vi "GTcode_v6.vi"() -> ()   [LabVIEW 2016]
uses:
  <vilib>/Utility/config.llb/Write Key (String).vi
  <vilib>/Utility/config.llb/Write Key (U32).vi
  <vilib>/Utility/config.llb/Write Key (Double).vi
  <vilib>/Utility/config.llb/Write Key (I32).vi
  <vilib>/Utility/config.llb/Read Key (U32).vi
  <vilib>/Utility/config.llb/Read Key (I32).vi
  DCScode_simulISS_MAP/flex05-4chPascal.dll
  <vilib>/Utility/config.llb/NI_LVConfig.lvlib
  DCScode_simulISS_MAP/flex05oem8chauto100nsPASCAL_win7.dll
  <vilib>/Analysis/NI_AALBase.lvlib
panel:
  in  "Tab Control":T1(tab)=enum."Real Time Fitting Parameters"
  out "mean":dbl format="%0.1e"
  out "COV":dbl format="%0.1f"
  in  "Fixed Time":bool
  in  "Detector Used":T2(ring)=enum."Det 2"
  in  "Real Time Fitting?":bool=TRUE
  out "g2":cluster{"Delay Time":sgl[], sgl[]}[](graph) caption="Normalized Correlation Function"
  out "Tau":cluster{"tmp":dbl, dbl}(graph) caption="Relative Changes of Flow"
  in  "QUIT":bool
  in  "Clear plots":bool
  in  "Baseline":bool
  in  "MARK\nMark":bool
  in  "Stop":bool
  in  "Sequence Scan":bool
  out "Mark #":u32
  out "Trial #":u32
  out "Frame #":u32
  out "Det 8":sgl format="%.3f"
  out "Det 7":sgl format="%.3f"
  out "Det 6":sgl format="%.3f"
  out "Det 5":sgl format="%.3f"
  out "Det 4":sgl format="%.3f"
  out "Det 3":sgl format="%.3f"
  out "Det 2":sgl format="%.3f"
  out "Det 1":sgl format="%.3f"
  out "Computer Time":string="2010-1-12 23:16:10"
  in  "D1":bool
  in  "D2":bool
  in  "D3":bool
  in  "D4":bool
  in  "D5":bool
  in  "D6":bool
  in  "D7":bool
  in  "D8":bool
  out "Tau 2":T3(graph)={1.6593152555505744e-08, 3.9427894777554196e-08, 4.065716407938411e-08, 1.5135790977358522e-08, 2.4870420100428357e-08, 7.094765128107397e-08, 0.0, 4.1348620928852906e-07, 1.5886917674344795e-08, 4.0280526032721455e-08, -1.0, -1.0} caption="Blood Flow Index (cm2/s)"
  in  "Fixed # of Frames":u32=5
  out "Status":string="Quit"
  in  "Optical Switch OPEN":bool
  in  "Delay between frames(ms)":u32=500
  out "Time Left (ms)":sgl format="%.3f"
  in  "Integration Time (ms)":sgl=1000.0 min=1 max=13000 step=1
  in  "File\nName:":string="test0"
  in  "Data Save Directory:":path=path "C:/data"
  in  "ISS Lasers ON":bool
  in  "Test":bool
  in  "Lines":tag="Dev1/port1/line0:1, Dev1/port1/line3:7"
  in  "Delaytime(ms)":u32=200
  in  "Initialize Correlator":bool
  in  "Detector Select":enum32{"4 Detectors", "8 Detectors"}(radio)=enum."8 Detectors"
  in  "Update Time (ms)\nDO NOT CHANGE!":u32=105 min=1 max=999 step=1
  in  "Laser Input Name":refnum<visa-resource-name>="COM7"
  out "Flow in each detector":dbl[](array[numeric])=[-1.0, -1.0, -1.0, -1.0, -1.0, -1.0, -1.0, -1.0, -1.0, -1.0, -1.0, -1.0]
  in  "Visible Averages":bool[](array[boolean])=[FALSE, FALSE, FALSE, FALSE]
  in  "Avg":bool[][](array[boolean])=[[FALSE, FALSE, FALSE, FALSE, FALSE, FALSE, FALSE, FALSE], [FALSE, FALSE, FALSE, FALSE, FALSE, FALSE, FALSE, FALSE], [FALSE, FALSE, FALSE, FALSE, FALSE, FALSE, FALSE, FALSE], [FALSE, FALSE, FALSE, FALSE, FALSE, FALSE, FALSE, FALSE]]
  in  "rho":dbl[](array[numeric])=[2.5, 2.5, 2.5, 2.5, 2.5, 2.5, 2.5, 2.5, -1.0, -1.0, -1.0, -1.0]
  in  "Other Settings":u32[](array[numeric])=[1, 120, 0, 1] caption="Flow in each detector"
  in  "Initial Guess":dbl[](array[numeric])=[1e-08, 0.5, 0.05, 10.0] caption="Flow in each detector"
  out "4CH?":bool
  out "Detector#":u32=1
  out "Source#":u32=1
  # "kHz"
  # "kHz"
  # "Don't Change these Parameters unless you know clearly what you are doing"
  # "ISS Triggers Setup"
  # "Channel Parameters"
  # "Step1"
  # "Line"
  # "0"
  # "1"
  # "3"
  # "4"
  # "5"
  # "6"
  # "7"
  # "*The number of lines in the list must\nmatch the number of elements in\nthe array."
  # "Step2"
  # "Line"
  # "0"
  # "1"
  # "3"
  # "4"
  # "5"
  # "6"
  # "7"
  # "Step3"
  # "Line"
  # "0"
  # "1"
  # "3"
  # "4"
  # "5"
  # "6"
  # "7"
  # "Line    Signal\n\n0           ISS Trigger (0: OFF, 1: ON)\n1           Flow Laser 1 ON/OFF (0:OFF, 1:ON)\n2           ISS Data Acquisition (0: DONE, 1: NO)\n3           ISS Laser ON/OFF (0: ON, 1: OFF)\n4           Trigger for Marks  (0: OFF, 1: ON)\n5           Flow Laser 2 ON/OFF (0:OFF, 1:ON)\n6           Reserved\n7           Reserved"
  # "Wait ISS Data Acuisition DONE Signal"
  # "Step4"
  # "Step5"
  # "Line"
  # "0"
  # "1"
  # "3"
  # "4"
  # "5"
  # "6"
  # "7"
  # "Flow Lasers Setup"
  # "FROM FRONT PANEL"
  # "Line"
  # "0"
  # "1"
  # "3"
  # "4"
  # "5"
  # "6"
  # "7"
  # "Line"
  # "0"
  # "1"
  # "3"
  # "4"
  # "5"
  # "6"
  # "7"
  # "Det 1"
  # "Det 2"
  # "Det 3"
  # "Det 4"
  # "Det 5"
  # "Det 6"
  # "Det 7"
  # "Det 8"
  # "Avg 1"
  # "Avg 2"
  # "Avg 3"
  # "Avg 4"
  # "Db"
  # "Beta"
  # "Mua"
  # "MuS'"
  # "1"
  # "2"
  # "3"
  # "4"
  # "5"
  # "6"
  # "7"
  # "8"
  # "Avg 1"
  # "Starting Pt"
  # "End Pt"
  # "Approximate"
  # "Variables"
  # "Avg 2"
  # "Avg 3"
  # "Avg 4"
  # "Source Detector  Separations"
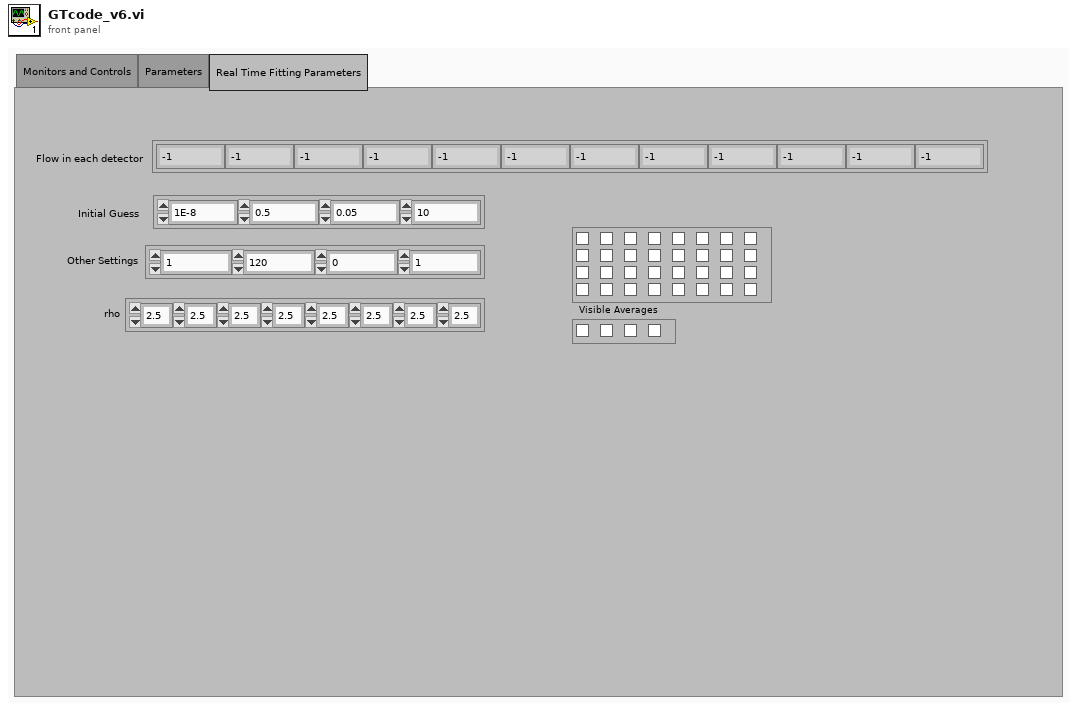
[diagram p1: front panel]
types:
  T1 = enum32{"Monitors and Controls", "Parameters", "Real Time Fitting Parameters"}
  T2 = enum16{"Det 1", "Det 2", "Det 3", "Det 4", "Det 5", "Det 6", "Det 7", "Det 8"}
  T3 = cluster{dbl, dbl, dbl, dbl, dbl, dbl, dbl, dbl, dbl, dbl, dbl, dbl}
  T4 = enum8{"Enabled", "Disabled", "Disabled and Grayed Out"}
  T5 = cluster{dbl, dbl, dbl, dbl, dbl, dbl, dbl, dbl, dbl, dbl, dbl, dbl}[]
  T6 = typedef "NI_LVConfig.lvlib/Config Data RefNum.ctl" = refnum<k1>
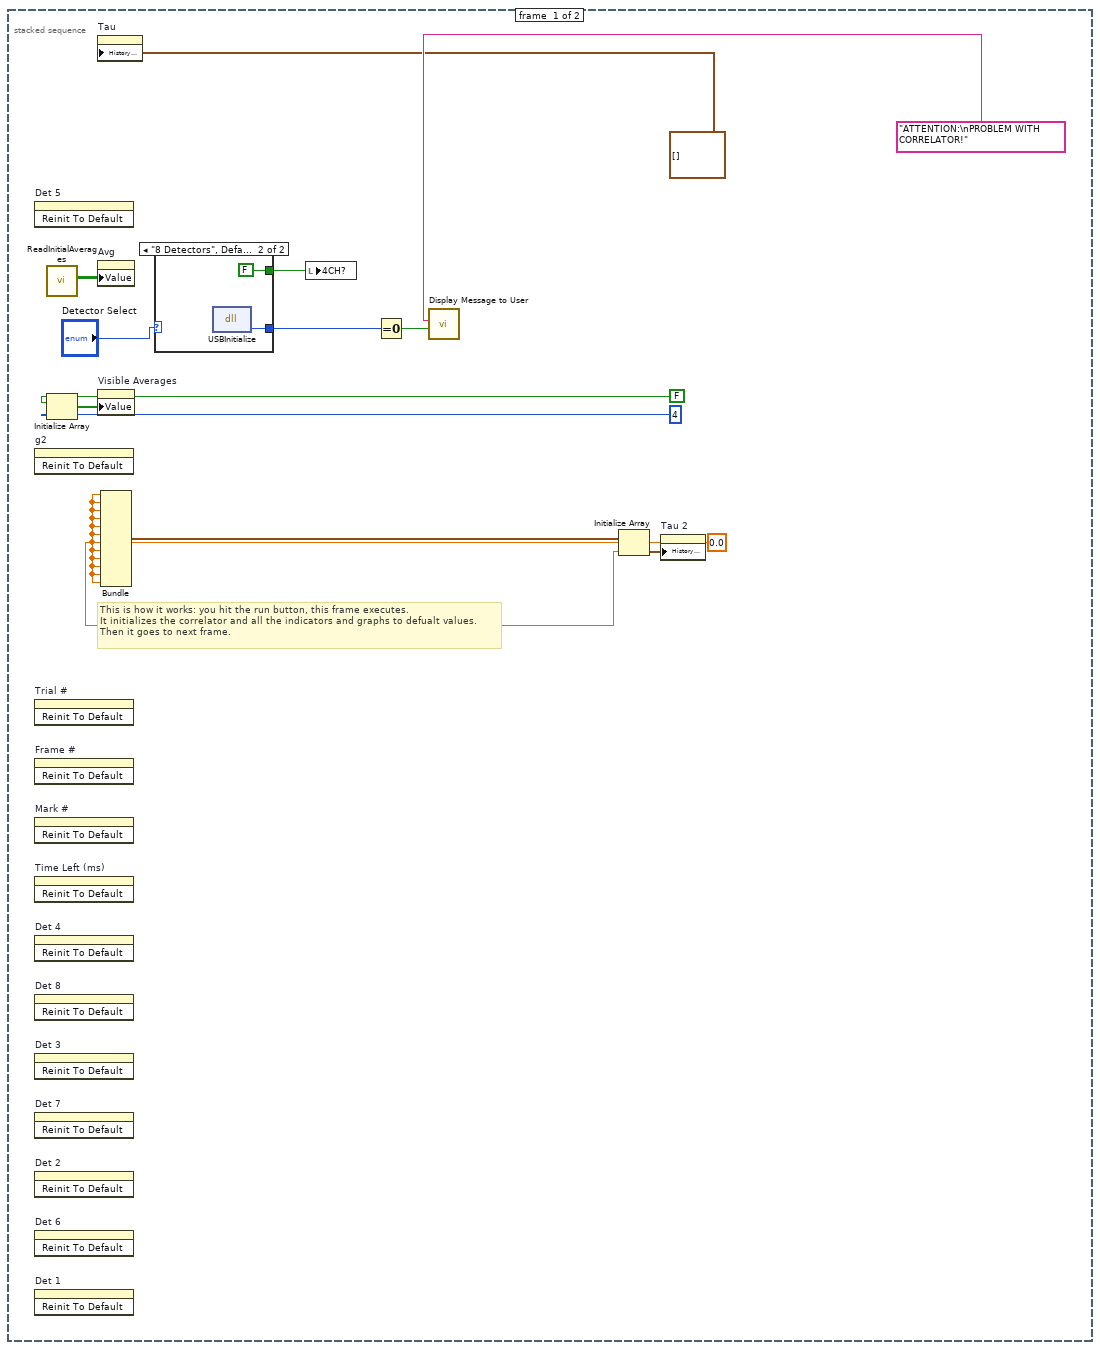
[diagram p2: hidden frame]
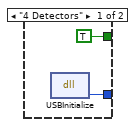
[diagram p3: hidden frame]
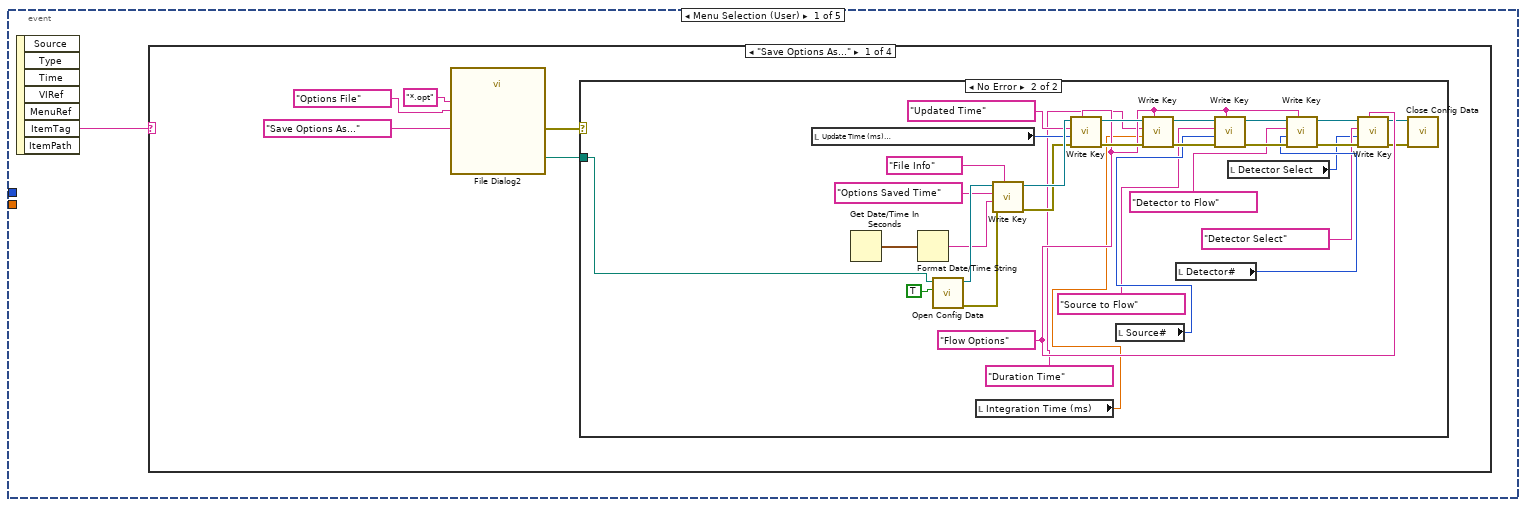
[diagram p5: hidden frame]
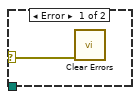
[diagram p6: hidden frame]
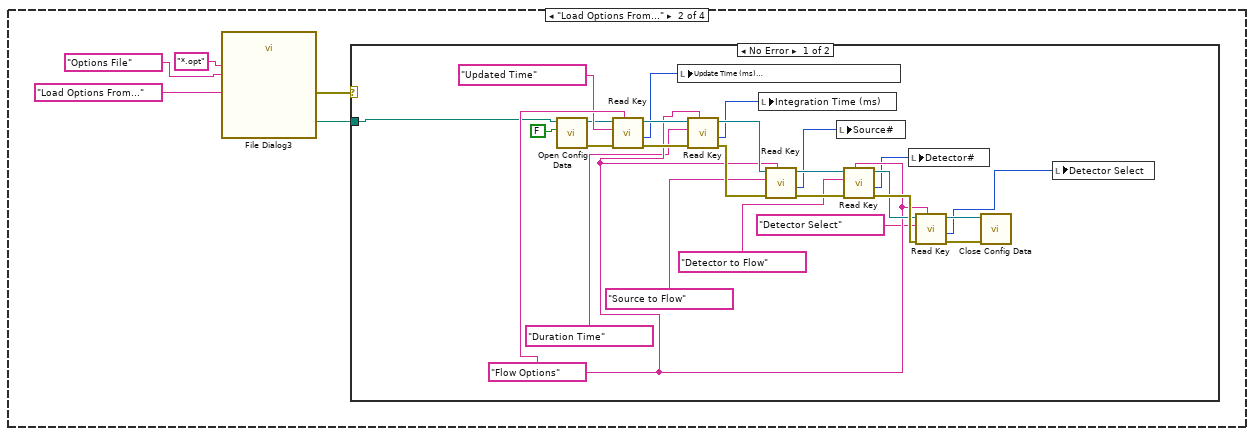
[diagram p7: hidden frame]
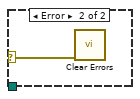
[diagram p8: hidden frame]
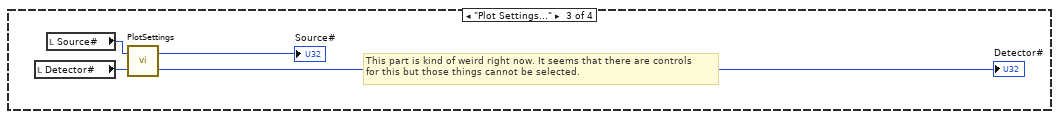
[diagram p9: hidden frame]
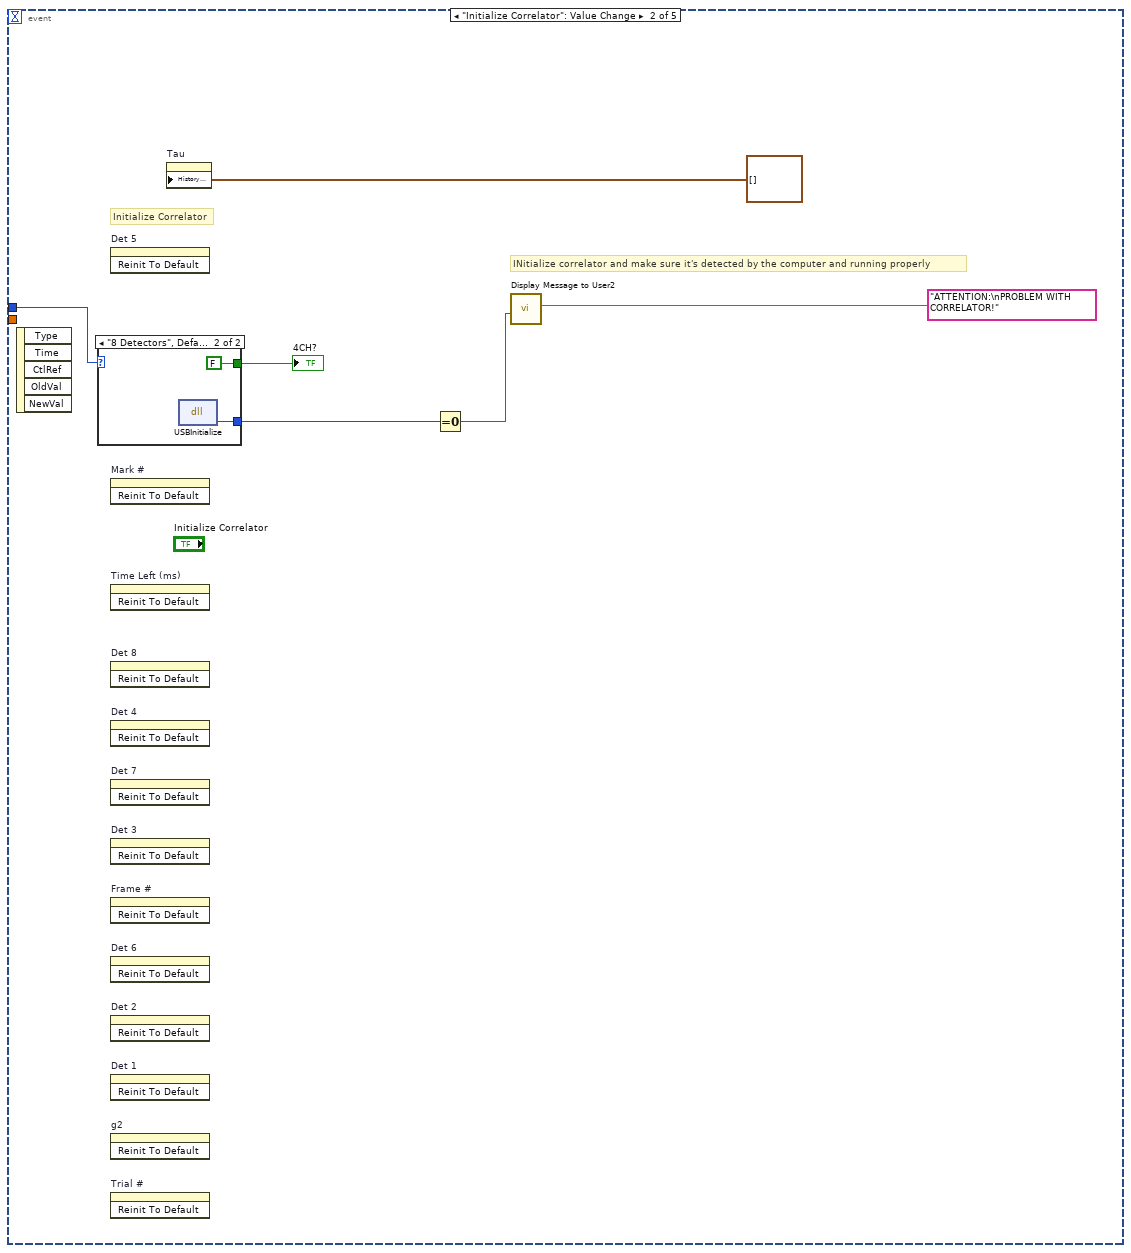
[diagram p11: hidden frame]
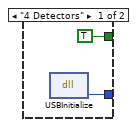
[diagram p12: hidden frame]
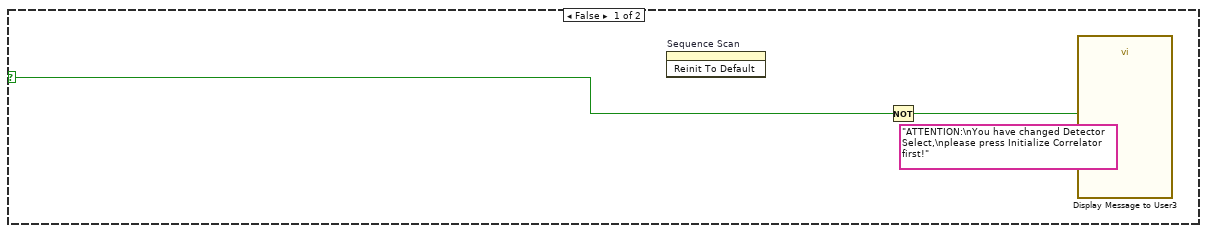
[diagram p13: hidden frame]
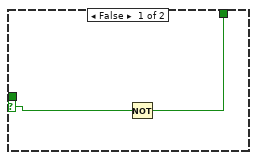
[diagram p14: hidden frame]
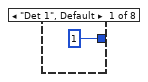
[diagram p20: hidden frame]
diagram:
  n1 = local read "Laser Input Name"() -> (w1:refnum<visa-resource-name>)
  n2 = call "iBs.vi"("Laser On/Off"=FALSE, "VISA resource name"=w1) -> ()
  n3 = stacked-sequence {
    frame #0 {
      w5 = 0.0
      # "This is how it works: you hit the run button, this frame executes.\nIt initializes the correlator and all the indicators and graphs to defualt values.\nThen it goes to next frame."
      n4 = invoke on="Det 5" class="DigNum (strict)" method="Reinit To Default"() -> ()  [unwired: 3 in, 3 out]
      n5 = invoke on="g2" class="XYGraph (strict)" method="Reinit To Default"() -> ()  [unwired: 3 in, 3 out]
      n6 = invoke on="Trial #" class="DigNum (strict)" method="Reinit To Default"() -> ()  [unwired: 3 in, 3 out]
      n7 = invoke on="Frame #" class="DigNum (strict)" method="Reinit To Default"() -> ()  [unwired: 3 in, 3 out]
      n8 = invoke on="Mark #" class="DigNum (strict)" method="Reinit To Default"() -> ()  [unwired: 3 in, 3 out]
      n9 = invoke on="Time Left (ms)" class="DigNum (strict)" method="Reinit To Default"() -> ()  [unwired: 3 in, 3 out]
      n10 = invoke on="Det 4" class="DigNum (strict)" method="Reinit To Default"() -> ()  [unwired: 3 in, 3 out]
      n11 = invoke on="Det 8" class="DigNum (strict)" method="Reinit To Default"() -> ()  [unwired: 3 in, 3 out]
      n12 = invoke on="Det 3" class="DigNum (strict)" method="Reinit To Default"() -> ()  [unwired: 3 in, 3 out]
      n13 = invoke on="Det 7" class="DigNum (strict)" method="Reinit To Default"() -> ()  [unwired: 3 in, 3 out]
      n14 = invoke on="Det 2" class="DigNum (strict)" method="Reinit To Default"() -> ()  [unwired: 3 in, 3 out]
      n15 = invoke on="Det 6" class="DigNum (strict)" method="Reinit To Default"() -> ()  [unwired: 3 in, 3 out]
      n16 = invoke on="Det 1" class="DigNum (strict)" method="Reinit To Default"() -> ()  [unwired: 3 in, 3 out]
      n17 = call "ReadInitialAverages.vi"() -> ("avgOut"=w4:bool[][])  [unwired: 11 in]
      n18 = Initialize Array(FALSE, 4) -> (w3:bool[])
      n19 = property on="Tau" class="WFChart (strict)"("History Data"=cluster{"tmp":dbl, dbl}[] []) -> ()  [unwired: 2 in, 2 out]
      n20 = property on="Avg" class="Arr (strict)"("Value"=w4) -> ()  [unwired: 2 in, 2 out]
      n21 = property on="Visible Averages" class="Arr (strict)"("Value"=w3) -> ()  [unwired: 2 in, 2 out]
      n22 = Bundle(w5, w5, w5, w5, w5, w5, w5, w5, w5, w5, w5, w5) -> (w7:T3)  [unwired: 1 in]
      n23 = case shown="\"8 Detectors\", Default" "Detector Select" {
        tunnel: [w17 w19] -> w15
        tunnel: [TRUE FALSE] -> w13
        frame "4 Detectors" {
          n24 = dll-call lib="C:/Users/BUCKLEY-ADMIN/Desktop/DCScode_simulISS_MAP/flex05-4chPascal.dll" fn="USBInitialize" label="InitCH4"() -> ("return type"=w17:u8)  [unwired: 3 in, 2 out]
        }
        frame "8 Detectors", Default {
          n25 = dll-call lib="C:/Users/BUCKLEY-ADMIN/Desktop/DCScode_simulISS_MAP/flex05oem8chauto100nsPASCAL_win7.dll" fn="USBInitialize" label="InitCH8"() -> ("return type"=w19:u8)  [unwired: 3 in, 2 out]
        }
      }
      n26 = local write "4CH?"(w13) -> ()
      n27 = Equal To 0?(x=w15) -> (x = 0?=w14:bool)
      n28 = call "Display Message to User"("Enable"=w14, "Message"="ATTENTION:\nPROBLEM WITH CORRELATOR!") -> ()  [unwired: 8 in, 2 out]
      n29 = Initialize Array(w7, w5) -> (w6:T5)
      n30 = property on="Tau 2" class="WFChart (strict)"("History Data"=w6) -> ()  [unwired: 2 in, 2 out]
    }
    frame #1 {
      n31 = while {
        stop <- w23 stop-if-true
        # "Looks at whether using 4 or 8 ch correlator\nGenerates time points for g2 function based on correlator"
        n32 = local read "Detector Select"() -> (w21:enum32{"4 Detectors", "8 Detectors"})
        n33 = case shown="\"8 Detectors\"" w21 {
          tunnel: [_ w24] -> w20
          frame "4 Detectors", Default {
          }
          frame "8 Detectors" {
            n34 = formula code="int i,j;\nfloat DelayTime[256];\nfloat first_delay;\n\nfirst_delay = 2E-7;\n\nfor(i=0;i<16;i++)\nDelayTime[i] = (i+1)*first_delay;\nfor(j=1;j<31;j++)\n    for(i=0;i<8;i++)\n         DelayTime[i+(j-1)*8+16] = DelayTime[(j-1)*8+16+i-1]+first_delay*pow(2,j);"() -> ("DelayTime"=w24:dbl[])
          }
        }
        n35 = event shown="[2] \"Sequence Scan\": Value Change" {
          selector: _ -> [_ _ _ _ _]
          dyn-events: _ -> [_ _ _ _ _]
          timeout: 500 -> [_ _ _ _ _]
          tunnel: w20 -> [_ _ w114 _ _]
          tunnel: [_ _ _ "QUIT" _] -> w23
          tunnel: w21 -> [_ w101 w110 w598 _]
          event Menu Selection (User) {
            n36 = event-data() -> ("ItemTag"=w25:string)  [unwired: 1 in, 6 out]
            n37 = case shown="\"Save Options As...\"" w25 {
              frame "Save Options As..." {
                n38 = call "File Dialog2"("prompt"="Save Options As...", "pattern (all files)"="*.opt", "pattern label"="Options File") -> ("selected path"=w27:path, "error out"=w26:errorcluster)  [unwired: 9 in, 2 out]
                n39 = case shown="No Error" w26 {
                  selector: w26 -> [w31 _]
                  tunnel: w27 -> [_ w62]
                  frame Error {
                    n40 = call <vilib>:"Clear Errors.vi"("error in (no error)"=w31) -> ()  [unwired: 5 in, 2 out]
                  }
                  frame No Error {
                    w49 = "Flow Options"
                    n41 = local read "Update Time (ms)\nDO NOT CHANGE!"() -> (w42:u32)
                    n42 = Get Date/Time In Seconds() -> (seconds since 1Jan1904=w48:timestamp)
                    n43 = Format Date/Time String(seconds (now)=w48) -> (date/time string=w44:string)  [unwired: 2 in]
                    n44 = call <vilib>:"Open Config Data.vi"("create file if necessary (T)"=TRUE, "configuration file path"=w62) -> ("error out"=w60:errorcluster, "refnum"=w59:T6)  [unwired: 7 in, 1 out]
                    n45 = local read "Integration Time (ms)"() -> (w40:sgl)
                    n46 = call-poly <vilib>:"Write Key.vi"("section"="File Info", "error in (no error)"=w60, "value"=w44, "key"="Options Saved Time", "refnum"=w59) -> ("error out"=w46:errorcluster, "refnum out"=w47:T6)  [unwired: 4 in, 1 out]
                    n47 = call-poly <vilib>:"Write Key.vi"("section"=w49, "error in (no error)"=w46, "value"=w42, "key"="Updated Time", "refnum"=w47) -> ("error out"=w58:errorcluster, "refnum out"=w57:T6)  [unwired: 4 in, 1 out]
                    n48 = local read "Source#"() -> (w39:u32)
                    n49 = call-poly <vilib>:"Write Key.vi"("section"=w49, "error in (no error)"=w58, "value"=w40, "key"="Duration Time", "refnum"=w57) -> ("error out"=w53:errorcluster, "refnum out"=w54:T6)  [unwired: 4 in, 1 out]
                    n50 = local read "Detector#"() -> (w36:u32)
                    n51 = call-poly <vilib>:"Write Key.vi"("section"=w49, "error in (no error)"=w53, "value"=w39, "key"="Source to Flow", "refnum"=w54) -> ("error out"=w55:errorcluster, "refnum out"=w56:T6)  [unwired: 4 in, 1 out]
                    n52 = local read "Detector Select"() -> (w34:enum32{"4 Detectors", "8 Detectors"})
                    n53 = call-poly <vilib>:"Write Key.vi"("section"=w49, "error in (no error)"=w55, "value"=w36, "key"="Detector to Flow", "refnum"=w56) -> ("error out"=w52:errorcluster, "refnum out"=w51:T6)  [unwired: 4 in, 1 out]
                    n54 = call-poly <vilib>:"Write Key.vi"("section"=w49, "error in (no error)"=w52, "value"=w34, "key"="Detector Select", "refnum"=w51) -> ("error out"=w32:errorcluster, "refnum out"=w33:T6)  [unwired: 4 in, 1 out]
                    n55 = call <vilib>:"Close Config Data.vi"("error in (no error)"=w32, "refnum"=w33) -> ()  [unwired: 8 in, 2 out]
                  }
                }
              }
              frame "Load Options From..." {
                n56 = call "File Dialog3"("prompt"="Load Options From...", "pattern (all files)"="*.opt", "pattern label"="Options File") -> ("selected path"=w64:path, "error out"=w63:errorcluster)  [unwired: 9 in, 2 out]
                n57 = case shown="No Error" w63 {
                  selector: w63 -> [_ w93]
                  tunnel: w64 -> [w68 _]
                  frame No Error {
                    w83 = "Flow Options"
                    n58 = call <vilib>:"Open Config Data.vi"("create file if necessary (T)"=FALSE, "configuration file path"=w68) -> ("error out"=w75:errorcluster, "refnum"=w74:T6)  [unwired: 7 in, 1 out]
                    n59 = call-poly <vilib>:"Read Key.vi"("section"=w83, "error in (no error)"=w75, "key"="Updated Time", "refnum"=w74) -> ("error out"=w91:errorcluster, "value"=w73:u32, "refnum out"=w90:T6)  [unwired: 4 in, 1 out]
                    n60 = local write "Update Time (ms)\nDO NOT CHANGE!"(w73) -> ()
                    n61 = call-poly <vilib>:"Read Key.vi"("section"=w83, "error in (no error)"=w91, "key"="Duration Time", "refnum"=w90) -> ("error out"=w86:errorcluster, "value"=w72:i32, "refnum out"=w87:T6)  [unwired: 4 in, 1 out]
                    n62 = local write "Integration Time (ms)"(w72) -> ()
                    n63 = call-poly <vilib>:"Read Key.vi"("section"=w83, "error in (no error)"=w86, "key"="Source to Flow", "refnum"=w87) -> ("error out"=w88:errorcluster, "value"=w69:u32, "refnum out"=w89:T6)  [unwired: 4 in, 1 out]
                    n64 = local write "Source#"(w69) -> ()
                    n65 = call-poly <vilib>:"Read Key.vi"("section"=w83, "error in (no error)"=w88, "key"="Detector to Flow", "refnum"=w89) -> ("error out"=w85:errorcluster, "value"=w70:u32, "refnum out"=w84:T6)  [unwired: 4 in, 1 out]
                    n66 = local write "Detector#"(w70) -> ()
                    n67 = call-poly <vilib>:"Read Key.vi"("section"=w83, "error in (no error)"=w85, "key"="Detector Select", "refnum"=w84) -> ("error out"=w76:errorcluster, "value"=w71:u32, "refnum out"=w77:T6)  [unwired: 4 in, 1 out]
                    n68 = call <vilib>:"Close Config Data.vi"("error in (no error)"=w76, "refnum"=w77) -> ()  [unwired: 8 in, 2 out]
                    n69 = local write "Detector Select"(w71) -> ()
                  }
                  frame Error {
                    n70 = call <vilib>:"Clear Errors.vi"("error in (no error)"=w93) -> ()  [unwired: 5 in, 2 out]
                  }
                }
              }
              frame "Plot Settings..." {
                # "This part is kind of weird right now. It seems that there are controls\nfor this but those things cannot be selected."
                n71 = local read "Detector#"() -> (w95:u32)
                n72 = local read "Source#"() -> (w96:u32)
                n73 = call "PlotSettings.vi"("Detectorin"=w95, "Sourcein"=w96) -> ("Detector#"=→"Detector#":u32, "Source#"=→"Source#":u32)
              }
              frame Default {
              }
            }
          }
          event "Initialize Correlator": Value Change {
            # "INitialize correlator and make sure it's detected by the computer and running properly"
            # "Initialize Correlator"
            n74 = event-data() -> ()  [unwired: 1 in, 5 out]
            n75 = case shown="\"8 Detectors\", Default" w101 {
              tunnel: [w105 w107] -> w103
              tunnel: [TRUE FALSE] -> w100
              frame "4 Detectors" {
                n76 = dll-call lib="C:/Users/BUCKLEY-ADMIN/Desktop/DCScode_simulISS_MAP/flex05-4chPascal.dll" fn="USBInitialize" label="InitCH4"() -> ("return type"=w105:u8)  [unwired: 3 in, 2 out]
              }
              frame "8 Detectors", Default {
                n77 = dll-call lib="C:/Users/BUCKLEY-ADMIN/Desktop/DCScode_simulISS_MAP/flex05oem8chauto100nsPASCAL_win7.dll" fn="USBInitialize" label="InitCH8"() -> ("return type"=w107:u8)  [unwired: 3 in, 2 out]
              }
            }
            "4CH?" <- w100
            n78 = invoke on="Det 5" class="DigNum (strict)" method="Reinit To Default"() -> ()  [unwired: 3 in, 3 out]
            n79 = invoke on="Mark #" class="DigNum (strict)" method="Reinit To Default"() -> ()  [unwired: 3 in, 3 out]
            n80 = invoke on="Time Left (ms)" class="DigNum (strict)" method="Reinit To Default"() -> ()  [unwired: 3 in, 3 out]
            n81 = invoke on="Det 8" class="DigNum (strict)" method="Reinit To Default"() -> ()  [unwired: 3 in, 3 out]
            n82 = invoke on="Det 4" class="DigNum (strict)" method="Reinit To Default"() -> ()  [unwired: 3 in, 3 out]
            n83 = invoke on="Det 7" class="DigNum (strict)" method="Reinit To Default"() -> ()  [unwired: 3 in, 3 out]
            n84 = invoke on="Det 3" class="DigNum (strict)" method="Reinit To Default"() -> ()  [unwired: 3 in, 3 out]
            n85 = invoke on="Frame #" class="DigNum (strict)" method="Reinit To Default"() -> ()  [unwired: 3 in, 3 out]
            n86 = invoke on="Det 6" class="DigNum (strict)" method="Reinit To Default"() -> ()  [unwired: 3 in, 3 out]
            n87 = invoke on="Det 2" class="DigNum (strict)" method="Reinit To Default"() -> ()  [unwired: 3 in, 3 out]
            n88 = invoke on="Det 1" class="DigNum (strict)" method="Reinit To Default"() -> ()  [unwired: 3 in, 3 out]
            n89 = invoke on="g2" class="XYGraph (strict)" method="Reinit To Default"() -> ()  [unwired: 3 in, 3 out]
            n90 = invoke on="Trial #" class="DigNum (strict)" method="Reinit To Default"() -> ()  [unwired: 3 in, 3 out]
            n91 = property on="Tau" class="WFChart (strict)"("History Data"=cluster{"tmp":dbl, dbl}[] []) -> ()  [unwired: 2 in, 2 out]
            n92 = Equal To 0?(x=w103) -> (x = 0?=w102:bool)
            n93 = call "Display Message to User2"("Enable"=w102, "Message"="ATTENTION:\nPROBLEM WITH CORRELATOR!") -> ()  [unwired: 8 in, 2 out]
          }
          event "Sequence Scan": Value Change {
            # "Initialize Baseline"
            n94 = event-data() -> ()  [unwired: 1 in, 6 out]
            n95 = case shown="\"8 Detectors\", Default" w110 {
              tunnel: [w593 w594] -> w109
              frame "4 Detectors" {
                n96 = local read "4CH?"() -> (w593:bool)
              }
              frame "8 Detectors", Default {
                # "Select whether using 4 or 8ch correlator"
                n97 = local read "4CH?"() -> (w595:bool)
                n98 = Not(x=w595) -> (.not. x?=w594:bool)
              }
            }
            n99 = case shown="True" w109 {
              selector: w109 -> [w116 _]
              tunnel: w114 -> [_ w130]
              tunnel: w110 -> [_ w131]
              tunnel: sgl 1.0 -> [_ w129]
              frame False {
                n100 = invoke on="Sequence Scan" class="Bool" method="Reinit To Default"() -> ()  [unwired: 3 in, 3 out]
                n101 = Not(x=w116) -> (.not. x?=w115:bool)
                n102 = call "Display Message to User3"("Enable"=w115, "Message"="ATTENTION:\nYou have changed Detector Select,\nplease press Initialize Correlator first!") -> ()  [unwired: 8 in, 2 out]
              }
              frame True {
                # "This part pauses and alerts user that test function is on. If test function is accepted then code runs but data is not saved (no timestamp either)."
                # "This checks for if the file already exists in the directory using the timing file. \n*If YES, then we don't do anything to the lasers. We just display message and wait for the user to input a new name and press sequence again.\n*If NO, then we proceed as per normal."
                n103 = local read "File\nName:"() -> (w125:string)
                n104 = case shown="True" "Test" {
                  selector: "Test" -> [w133 _]
                  tunnel: "Test" -> [_ w135]
                  tunnel: [w132 w134] -> w118
                  frame False {
                    n105 = Not(x=w133) -> (.not. x?=w132:bool)
                  }
                  frame True {
                    n106 = call "Test ON"("Enable"=w135) -> ("No - STOP"=w136:bool, "OK"=w134:bool)  [unwired: 15 in, 2 out]
                    n107 = local write "Stop"(w136) -> ()
                  }
                }
                n108 = local read "Data Save Directory:"() -> (w124:path)
                n109 = Concatenate Strings(w125, "_TIMING", ".dat") -> (w127:string)
                n110 = Build Path(base path=w124, name or relative path=w127) -> (appended path=w123:path)
                n111 = call <vilib>:"Check if File or Folder Exists.vi"("path"=w123) -> ("file or folder exists?"=w120:bool)  [unwired: 8 in, 2 out]
                n112 = Not(x=w120) -> (.not. x?=w122:bool)
                n113 = Not And(1:w118, 2:w122) -> (0:w121:bool)
                n114 = case shown="False" w121 {
                  tunnel: w131 -> [w150 _]
                  tunnel: w130 -> [w149 _]
                  tunnel: w129 -> [w148 _]
                  frame False {
                    # "Turn relay on so that Optical switch is open and LED indicator is ON"
                    # "When the START button is pressed, the ISS lasers turn off"
                    n115 = local read "Test"() -> (w137:bool)
                    n116 = case shown="False" w137 {
                      frame False {
                        # "This bit stores the time stamp."
                        n117 = local read "File\nName:"() -> (w151:string)
                        n118 = Get Date/Time In Seconds() -> (seconds since 1Jan1904=w153:timestamp)
                        n119 = local read "Data Save Directory:"() -> (w152:path)
                        n120 = Format Date/Time String(seconds (now)=w153) -> (date/time string=w159:string)  [unwired: 2 in]
                        n121 = Concatenate Strings(w151, "_TIMING", ".dat") -> (w156:string)
                        n122 = Build Path(base path=w152, name or relative path=w156) -> (appended path=w155:path)
                        n123 = Write to Text File(file (use dialog)=w155, text=w159) -> (refnum out=w158:refnum<file>, error out=w157:errorcluster)  [unwired: 2 in, 1 out]
                        n124 = Close File(refnum=w158, error in=w157) -> ()  [unwired: 2 out]
                      }
                      frame True {
                      }
                    }
                    n125 = Build Array(TRUE, TRUE) -> (w147:bool[])
                    n126 = Build Array(FALSE) -> (w144:bool[])
                    n127 = local read "Fixed # of Frames"() -> (w142:u32)
                    n128 = call "DAQ Assistant"("data"=w147) -> ()  [unwired: 17 in, 2 out]
                    n129 = call "DAQ Assistant7"("data"=w144) -> ()  [unwired: 17 in, 2 out]
                    n130 = Initialize Array "Initialize Array"(nan, w142) -> (w140:dbl[])
                    n131 = while {
                      tunnel: w150 -> [w194]
                      tunnel: w149 -> [w193]
                      tunnel: w148 -> [_]
                      shift-right: [w165] -> _
                      shift-left: w140 -> [w166]
                      stop <- w167 stop-if-true
                      # "Only runs Real Time Fitting if \nReal Time Fitting box is checked \nand test function is off."
                      # "After testing is complete, turn off the lasers and\nreset  the buttons."
                      n132 = for {
                        N: 1 -> [_]
                        tunnel: w193 -> [w235]
                        tunnel: w194 -> [w234]
                        tunnel: [w231] -> w167
                        tunnel: [w230] -> w191
                        tunnel: [w228] -> w171
                        tunnel: [w227] -> w170
                        tunnel: [w226] -> w169
                        # "The logic here may look funny but it works elegantly. No matter if you choose \"Use Both Lasers\", the AND output is always\nfalse the first time these two boxes run since Laser 1 Value is always false, and the default is to use flow laser 1.\nBUT, the trick is if you chose \"Use Both Laser\" This big for loop is gonna run twice, the second time it runs, \nthe laser 1 value is TRUE because it is set to TRUE by the second box when the big for loop ran the first time. Now, when\nthe output of AND is true, ISS laser no longer runs. Only flow laser two is turned on and we execute the for loop to the right."
                        # "These two boxes take care of the flow chart.\nIt turn on ISS laser first, then triggers it and turn it off.\nIf ISS data is ready, then we go on to flow lase."
                        # "This loop may seem useless but it acts as a block. \nThis block does all the data collection, plotting and writing the data\nto file"
                        n133 = case shown="\"8 Detectors\", Default" w234 {
                          selector: w234 -> [w591 w592]
                          tunnel: [w591 w592] -> w232
                          frame "4 Detectors" {
                            n134 = dll-call lib="C:/Users/BUCKLEY-ADMIN/Desktop/DCScode_simulISS_MAP/flex05-4chPascal.dll" fn="USBStart" label="StartCH4"() -> ()  [unwired: 4 in, 2 out]
                          }
                          frame "8 Detectors", Default {
                            n135 = dll-call lib="C:/Users/BUCKLEY-ADMIN/Desktop/DCScode_simulISS_MAP/flex05oem8chauto100nsPASCAL_win7.dll" fn="USBStart" label="StartCH8"() -> ()  [unwired: 4 in, 2 out]
                          }
                        }
                        n136 = for {
                          N: 1 -> [_]
                          tunnel: w235 -> [w256]
                          tunnel: [w240] -> w231
                          tunnel: w232 -> [w245]
                          tunnel: [w248] -> w230
                          tunnel: "MARK\nMark" -> [w247]
                          tunnel: [w246] -> w228
                          tunnel: [w237] -> w227
                          tunnel: [w244] -> w226
                          w257 = FALSE
                          w266 = u8 2
                          # "Only saves data if\ntest function is off."
                          # "If Fixed # Frames check box is selected,\ncode will run for # of frames specified on \nfront panel and then call Stop button"
                          # "This for loop here acts as a block as well. It takes the relative \nflow data from UpdateData.vi and plot the data on the graph.\nWhen \"Baseline\" is selected,  the data point goes to 1. When\n\"Mark\" is selected, a point at positive infinity is plotted and a\nvertical line joining the point and the x axis if displayed."
                          n137 = while {
                            tunnel: [w447] -> w265
                            tunnel: [w417] -> w264
                            tunnel: [w418] -> w263
                            tunnel: [w421] -> w240
                            tunnel: [w448] -> w262
                            tunnel: w256 -> [w450]
                            tunnel: w245 -> [w423]
                            stop <- w452 stop-if-true
                            # "D4 Tail Alarm"
                            # "D2 Tail Alarm"
                            # "D8 Tail Alarm"
                            # "D7 Tail Alarm"
                            # "D6 Tail Alarm"
                            # "D5 Tail Alarm"
                            # "D3 Tail Alarm"
                            # "D1 Tail Alarm"
                            # "When press STOP, turn off DCS laser LED indicator is OFF"
                            n138 = Not(x="D4") -> (.not. x?=w436:bool)
                            n139 = Not(x="D8") -> (.not. x?=w432:bool)
                            n140 = Not(x="D5") -> (.not. x?=w435:bool)
                            n141 = Not(x="D1") -> (.not. x?=w439:bool)
                            n142 = Not(x="D6") -> (.not. x?=w434:bool)
                            n143 = Not(x="D2") -> (.not. x?=w424:bool)
                            n144 = Not(x="D7") -> (.not. x?=w433:bool)
                            n145 = Not(x="D3") -> (.not. x?=w437:bool)
                            n146 = case shown="True" "Stop" {
                              selector: "Stop" -> [w491 w497]
                              tunnel: [w491 w494] -> w421
                              frame False {
                              }
                              frame True {
                                n147 = call "Prompt User for Input"("Enable"=w497) -> ("Yes"=w494:bool)  [unwired: 17 in, 1 out]
                                n148 = Build Array(w494, FALSE) -> (w496:bool[])
                                n149 = call "DAQ Assistant2"("data"=w496) -> ()  [unwired: 17 in, 2 out]
                                n150 = local read "Laser Input Name"() -> (w492:refnum<visa-resource-name>)
                                n151 = call "iBs.vi"("Laser On/Off"=FALSE, "VISA resource name"=w492) -> ()
                              }
                            }
                            n152 = case shown="True" "Clear plots" {
                              frame False {
                              }
                              frame True {
                                n153 = invoke on="g2" class="XYGraph (strict)" method="Reinit To Default"() -> ()  [unwired: 3 in, 3 out]
                              }
                            }
                            n154 = case shown="False" w436 {
                              selector: w436 -> [w538 w543]
                              frame False {
                                n155 = property on="Tau 2" class="WFChart (strict)"("Active Plot"=u32 3) -> (error out=w540:errorcluster)  [unwired: 2 in, 1 out]
                                n156 = property on="g2" class="XYGraph (strict)"("Active Plot"=u32 3) -> (error out=w541:errorcluster)  [unwired: 2 in, 1 out]
                                n157 = property on="g2" class="XYGraph (strict)"(error in=w541, "Plot.Visible?"=w538) -> ()  [unwired: 1 in, 2 out]
                                n158 = property on="Tau 2" class="WFChart (strict)"(error in=w540, "Plot.Visible?"=w538) -> ()  [unwired: 1 in, 2 out]
                              }
                              frame True {
                                n159 = property on="Tau 2" class="WFChart (strict)"("Active Plot"=u32 3) -> (error out=w544:errorcluster)  [unwired: 2 in, 1 out]
                                n160 = property on="Tau 2" class="WFChart (strict)"(error in=w544, "Plot.Visible?"=w543) -> ()  [unwired: 1 in, 2 out]
                                n161 = property on="g2" class="XYGraph (strict)"("Active Plot"=u32 3) -> (error out=w546:errorcluster)  [unwired: 2 in, 1 out]
                                n162 = property on="g2" class="XYGraph (strict)"(error in=w546, "Plot.Visible?"=w543) -> ()  [unwired: 1 in, 2 out]
                              }
                            }
                            n163 = case shown="False" w432 {
                              selector: w432 -> [w498 w503]
                              frame False {
                                n164 = property on="Tau 2" class="WFChart (strict)"("Active Plot"=u32 7) -> (error out=w499:errorcluster)  [unwired: 2 in, 1 out]
                                n165 = property on="g2" class="XYGraph (strict)"("Active Plot"=u32 7) -> (error out=w501:errorcluster)  [unwired: 2 in, 1 out]
                                n166 = property on="g2" class="XYGraph (strict)"(error in=w501, "Plot.Visible?"=w498) -> ()  [unwired: 1 in, 2 out]
                                n167 = property on="Tau 2" class="WFChart (strict)"(error in=w499, "Plot.Visible?"=w498) -> ()  [unwired: 1 in, 2 out]
                              }
                              frame True {
                                n168 = property on="Tau 2" class="WFChart (strict)"("Active Plot"=u32 7) -> (error out=w505:errorcluster)  [unwired: 2 in, 1 out]
                                n169 = property on="Tau 2" class="WFChart (strict)"(error in=w505, "Plot.Visible?"=w503) -> ()  [unwired: 1 in, 2 out]
                                n170 = property on="g2" class="XYGraph (strict)"("Active Plot"=u32 7) -> (error out=w506:errorcluster)  [unwired: 2 in, 1 out]
                                n171 = property on="g2" class="XYGraph (strict)"(error in=w506, "Plot.Visible?"=w503) -> ()  [unwired: 1 in, 2 out]
                              }
                            }
                            n172 = case shown="False" w435 {
                              selector: w435 -> [w528 w533]
                              frame False {
                                n173 = property on="Tau 2" class="WFChart (strict)"("Active Plot"=u32 4) -> (error out=w530:errorcluster)  [unwired: 2 in, 1 out]
                                n174 = property on="g2" class="XYGraph (strict)"("Active Plot"=u32 4) -> (error out=w531:errorcluster)  [unwired: 2 in, 1 out]
                                n175 = property on="g2" class="XYGraph (strict)"(error in=w531, "Plot.Visible?"=w528) -> ()  [unwired: 1 in, 2 out]
                                n176 = property on="Tau 2" class="WFChart (strict)"(error in=w530, "Plot.Visible?"=w528) -> ()  [unwired: 1 in, 2 out]
                              }
                              frame True {
                                n177 = property on="Tau 2" class="WFChart (strict)"("Active Plot"=u32 4) -> (error out=w535:errorcluster)  [unwired: 2 in, 1 out]
                                n178 = property on="Tau 2" class="WFChart (strict)"(error in=w535, "Plot.Visible?"=w533) -> ()  [unwired: 1 in, 2 out]
                                n179 = property on="g2" class="XYGraph (strict)"("Active Plot"=u32 4) -> (error out=w536:errorcluster)  [unwired: 2 in, 1 out]
                                n180 = property on="g2" class="XYGraph (strict)"(error in=w536, "Plot.Visible?"=w533) -> ()  [unwired: 1 in, 2 out]
                              }
                            }
                            n181 = case shown="False" w439 {
                              selector: w439 -> [w568 w573]
                              frame False {
                                n182 = property on="Tau 2" class="WFChart (strict)"("Active Plot"=u32 0) -> (error out=w569:errorcluster)  [unwired: 2 in, 1 out]
                                n183 = property on="g2" class="XYGraph (strict)"("Active Plot"=u32 0) -> (error out=w571:errorcluster)  [unwired: 2 in, 1 out]
                                n184 = property on="g2" class="XYGraph (strict)"(error in=w571, "Plot.Visible?"=w568) -> ()  [unwired: 1 in, 2 out]
                                n185 = property on="Tau 2" class="WFChart (strict)"(error in=w569, "Plot.Visible?"=w568) -> ()  [unwired: 1 in, 2 out]
                              }
                              frame True {
                                n186 = property on="Tau 2" class="WFChart (strict)"("Active Plot"=u32 0) -> (error out=w575:errorcluster)  [unwired: 2 in, 1 out]
                                n187 = property on="Tau 2" class="WFChart (strict)"(error in=w575, "Plot.Visible?"=w573) -> ()  [unwired: 1 in, 2 out]
                                n188 = property on="g2" class="XYGraph (strict)"("Active Plot"=u32 0) -> (error out=w576:errorcluster)  [unwired: 2 in, 1 out]
                                n189 = property on="g2" class="XYGraph (strict)"(error in=w576, "Plot.Visible?"=w573) -> ()  [unwired: 1 in, 2 out]
                              }
                            }
                            n190 = case shown="False" w434 {
                              selector: w434 -> [w518 w523]
                              frame False {
                                n191 = property on="Tau 2" class="WFChart (strict)"("Active Plot"=u32 5) -> (error out=w520:errorcluster)  [unwired: 2 in, 1 out]
                                n192 = property on="g2" class="XYGraph (strict)"("Active Plot"=u32 5) -> (error out=w521:errorcluster)  [unwired: 2 in, 1 out]
                                n193 = property on="g2" class="XYGraph (strict)"(error in=w521, "Plot.Visible?"=w518) -> ()  [unwired: 1 in, 2 out]
                                n194 = property on="Tau 2" class="WFChart (strict)"(error in=w520, "Plot.Visible?"=w518) -> ()  [unwired: 1 in, 2 out]
                              }
                              frame True {
                                n195 = property on="Tau 2" class="WFChart (strict)"("Active Plot"=u32 5) -> (error out=w524:errorcluster)  [unwired: 2 in, 1 out]
                                n196 = property on="Tau 2" class="WFChart (strict)"(error in=w524, "Plot.Visible?"=w523) -> ()  [unwired: 1 in, 2 out]
                                n197 = property on="g2" class="XYGraph (strict)"("Active Plot"=u32 5) -> (error out=w526:errorcluster)  [unwired: 2 in, 1 out]
                                n198 = property on="g2" class="XYGraph (strict)"(error in=w526, "Plot.Visible?"=w523) -> ()  [unwired: 1 in, 2 out]
                              }
                            }
                            n199 = case shown="False" w424 {
                              selector: w424 -> [w558 w563]
                              frame False {
                                n200 = property on="Tau 2" class="WFChart (strict)"("Active Plot"=u32 1) -> (error out=w560:errorcluster)  [unwired: 2 in, 1 out]
                                n201 = property on="g2" class="XYGraph (strict)"("Active Plot"=u32 1) -> (error out=w561:errorcluster)  [unwired: 2 in, 1 out]
                                n202 = property on="g2" class="XYGraph (strict)"(error in=w561, "Plot.Visible?"=w558) -> ()  [unwired: 1 in, 2 out]
                                n203 = property on="Tau 2" class="WFChart (strict)"(error in=w560, "Plot.Visible?"=w558) -> ()  [unwired: 1 in, 2 out]
                              }
                              frame True {
                                n204 = property on="Tau 2" class="WFChart (strict)"("Active Plot"=u32 1) -> (error out=w565:errorcluster)  [unwired: 2 in, 1 out]
                                n205 = property on="Tau 2" class="WFChart (strict)"(error in=w565, "Plot.Visible?"=w563) -> ()  [unwired: 1 in, 2 out]
                                n206 = property on="g2" class="XYGraph (strict)"("Active Plot"=u32 1) -> (error out=w566:errorcluster)  [unwired: 2 in, 1 out]
                                n207 = property on="g2" class="XYGraph (strict)"(error in=w566, "Plot.Visible?"=w563) -> ()  [unwired: 1 in, 2 out]
                              }
                            }
                            n208 = case shown="False" w433 {
                              selector: w433 -> [w508 w513]
                              frame False {
                                n209 = property on="Tau 2" class="WFChart (strict)"("Active Plot"=u32 6) -> (error out=w510:errorcluster)  [unwired: 2 in, 1 out]
                                n210 = property on="g2" class="XYGraph (strict)"("Active Plot"=u32 6) -> (error out=w511:errorcluster)  [unwired: 2 in, 1 out]
                                n211 = property on="g2" class="XYGraph (strict)"(error in=w511, "Plot.Visible?"=w508) -> ()  [unwired: 1 in, 2 out]
                                n212 = property on="Tau 2" class="WFChart (strict)"(error in=w510, "Plot.Visible?"=w508) -> ()  [unwired: 1 in, 2 out]
                              }
                              frame True {
                                n213 = property on="Tau 2" class="WFChart (strict)"("Active Plot"=u32 6) -> (error out=w514:errorcluster)  [unwired: 2 in, 1 out]
                                n214 = property on="Tau 2" class="WFChart (strict)"(error in=w514, "Plot.Visible?"=w513) -> ()  [unwired: 1 in, 2 out]
                                n215 = property on="g2" class="XYGraph (strict)"("Active Plot"=u32 6) -> (error out=w516:errorcluster)  [unwired: 2 in, 1 out]
                                n216 = property on="g2" class="XYGraph (strict)"(error in=w516, "Plot.Visible?"=w513) -> ()  [unwired: 1 in, 2 out]
                              }
                            }
                            n217 = case shown="False" w437 {
                              selector: w437 -> [w548 w553]
                              frame False {
                                n218 = property on="Tau 2" class="WFChart (strict)"("Active Plot"=u32 2) -> (error out=w549:errorcluster)  [unwired: 2 in, 1 out]
                                n219 = property on="g2" class="XYGraph (strict)"("Active Plot"=u32 2) -> (error out=w551:errorcluster)  [unwired: 2 in, 1 out]
                                n220 = property on="g2" class="XYGraph (strict)"(error in=w551, "Plot.Visible?"=w548) -> ()  [unwired: 1 in, 2 out]
                                n221 = property on="Tau 2" class="WFChart (strict)"(error in=w549, "Plot.Visible?"=w548) -> ()  [unwired: 1 in, 2 out]
                              }
                              frame True {
                                n222 = property on="Tau 2" class="WFChart (strict)"("Active Plot"=u32 2) -> (error out=w555:errorcluster)  [unwired: 2 in, 1 out]
                                n223 = property on="Tau 2" class="WFChart (strict)"(error in=w555, "Plot.Visible?"=w553) -> ()  [unwired: 1 in, 2 out]
                                n224 = property on="g2" class="XYGraph (strict)"("Active Plot"=u32 2) -> (error out=w556:errorcluster)  [unwired: 2 in, 1 out]
                                n225 = property on="g2" class="XYGraph (strict)"(error in=w556, "Plot.Visible?"=w553) -> ()  [unwired: 1 in, 2 out]
                              }
                            }
                            n226 = Wait (ms)(milliseconds to wait="Update Time (ms)\nDO NOT CHANGE!") -> ()  [unwired: 1 out]
                            n227 = call "UpdateData.vi"("Duration Time (ms)"="Integration Time (ms)", "Detector Select"=w423, "Delay Time"=w450) -> ("Elapsed Time(s)"=w451:sgl, "Intensity Array"=w449:sgl[], "Tau Array"=w448:sgl[], "mean"=w413:dbl, "mean 8"=w393:dbl, "mean 2"=w362:dbl, "mean 7"=w394:dbl, "mean 3"=w398:dbl, "Intensity data"=w447:string, "g2 Display"=→"g2":cluster{"Delay Time":sgl[], sgl[]}[], "mean 4"=w397:dbl, "mean 5"=w396:dbl, "mean 6"=w395:dbl, "tau data"=w417:string, "g2 data"=w418:string)  [unwired: 2 in]
                            n228 = Multiply(x=sgl 1000.0, y=w451) -> (x*y=w455:sgl)
                            n229 = Less?(x=w413, y=1.005) -> (x < y?=w392:bool)
                            n230 = Less?(x=w362, y=1.005) -> (x < y?=w346:bool)
                            n231 = Less?(x=w398, y=1.005) -> (x < y?=w345:bool)
                            n232 = Less?(x=w397, y=1.005) -> (x < y?=w342:bool)
                            n233 = Less?(x=w396, y=1.005) -> (x < y?=w340:bool)
                            n234 = Less?(x=w395, y=1.005) -> (x < y?=w338:bool)
                            n235 = Less?(x=w394, y=1.005) -> (x < y?=w336:bool)
                            n236 = Less?(x=w393, y=1.005) -> (x < y?=w334:bool)
                            n237 = Index Array(array=w449, index #1=0, index #2=1, index #3=2, index #4=3, index #5=4, index #6=5, index #7=6, index #8=7) -> (element #1=w390:sgl, element #2=w369:sgl, element #3=w368:sgl, element #4=w367:sgl, element #5=w366:sgl, element #6=w365:sgl, element #7=w364:sgl, element #8=w363:sgl)
                            "Det 7" <- w364
                            "Det 6" <- w365
                            "Det 5" <- w366
                            "Det 4" <- w367
                            "Det 3" <- w368
                            "Det 2" <- w369
                            "Det 1" <- w390
                            "Det 8" <- w363
                            n238 = Subtract(x="Integration Time (ms)", y=w455) -> (x-y=w453:sgl)
                            "Time Left (ms)" <- w453
                            n239 = Greater?(x=w413, y=0.98) -> (0:w391:bool)
                            n240 = Greater?(x=w397, y=0.98) -> (0:w343:bool)
                            n241 = Greater?(x=w395, y=0.98) -> (0:w339:bool)
                            n242 = Greater?(x=w393, y=0.98) -> (0:w335:bool)
                            n243 = Greater Or Equal?(x=w390, y=sgl 2.0) -> (x >= y?=w387:bool)
                            n244 = Greater Or Equal?(x=w369, y=sgl 2.0) -> (x >= y?=w333:bool)
                            n245 = Greater Or Equal?(x=w368, y=sgl 2.0) -> (x >= y?=w331:bool)
                            n246 = Greater Or Equal?(x=w367, y=sgl 2.0) -> (x >= y?=w329:bool)
                            n247 = Greater Or Equal?(x=w366, y=sgl 2.0) -> (x >= y?=w327:bool)
                            n248 = Greater Or Equal?(x=w365, y=sgl 2.0) -> (x >= y?=w325:bool)
                            n249 = Less Or Equal?(x=w390, y=sgl 1000.0) -> (x <= y?=w386:bool)
                            n250 = Less Or Equal?(x=w369, y=sgl 1000.0) -> (x <= y?=w332:bool)
                            n251 = Less Or Equal?(x=w368, y=sgl 1000.0) -> (x <= y?=w330:bool)
                            n252 = Less Or Equal?(x=w367, y=sgl 1000.0) -> (x <= y?=w328:bool)
                            n253 = Less Or Equal?(x=w366, y=sgl 1000.0) -> (x <= y?=w326:bool)
                            n254 = Less Or Equal?(x=w365, y=sgl 1000.0) -> (x <= y?=w324:bool)
                            n255 = Less Or Equal?(x=w364, y=sgl 1000.0) -> (x <= y?=w322:bool)
                            n256 = Less Or Equal?(x=w363, y=sgl 1000.0) -> (x <= y?=w320:bool)
                            n257 = Greater Or Equal?(x=w364, y=sgl 2.0) -> (x >= y?=w323:bool)
                            n258 = Greater Or Equal?(x=w363, y=sgl 2.0) -> (x >= y?=w321:bool)
                            n259 = Greater?(x=w362, y=0.98) -> (0:w347:bool)
                            n260 = Greater?(x=w398, y=0.98) -> (0:w344:bool)
                            n261 = Greater?(x=w396, y=0.98) -> (0:w341:bool)
                            n262 = Greater?(x=w394, y=0.98) -> (0:w337:bool)
                            n263 = Build Array(w392, w391, w387, w386) -> (w385:bool[])
                            n264 = Build Array(w347, w346, w333, w332) -> (w361:bool[])
                            n265 = Build Array(w345, w344, w331, w330) -> (w360:bool[])
                            n266 = Build Array(w343, w342, w329, w328) -> (w359:bool[])
                            n267 = Build Array(w341, w340, w327, w326) -> (w358:bool[])
                            n268 = Build Array(w339, w338, w325, w324) -> (w357:bool[])
                            n269 = Build Array(w337, w336, w323, w322) -> (w356:bool[])
                            n270 = Build Array(w335, w334, w321, w320) -> (w355:bool[])
                            n271 = And Array Elements(Boolean array=w385) -> (logical AND=w384:bool)
                            n272 = And Array Elements(Boolean array=w361) -> (logical AND=w348:bool)
                            n273 = And Array Elements(Boolean array=w360) -> (logical AND=w349:bool)
                            n274 = And Array Elements(Boolean array=w359) -> (logical AND=w350:bool)
                            n275 = And Array Elements(Boolean array=w358) -> (logical AND=w351:bool)
                            n276 = And Array Elements(Boolean array=w357) -> (logical AND=w352:bool)
                            n277 = And Array Elements(Boolean array=w356) -> (logical AND=w353:bool)
                            n278 = And Array Elements(Boolean array=w355) -> (logical AND=w354:bool)
                            n279 = Less Or Equal To 0?(x=w453) -> (x <= 0?=w454:bool)
                            n280 = case shown="True" w384 {
                              frame False {
                                n281 = control-ref of="Det 1"() -> (w487:refnum<vi>)
                                n282 = property on="Property Node" class="Digital (strict)"(reference=w487, "DisabledEnum"=T4."Disabled and Grayed Out" ("Disabled")) -> ()  [unwired: 1 in, 2 out]
                              }
                              frame True {
                                n283 = control-ref of="Det 1"() -> (w489:refnum<vi>)
                                n284 = property on="Property Node" class="Digital (strict)"(reference=w489, "DisabledEnum"=T4."Enabled" ("Disabled")) -> ()  [unwired: 1 in, 2 out]
                              }
                            }
                            n285 = case shown="True" w348 {
                              frame False {
                                n286 = control-ref of="Det 2"() -> (w483:refnum<vi>)
                                n287 = property on="Property Node" class="Digital (strict)"(reference=w483, "DisabledEnum"=T4."Disabled and Grayed Out" ("Disabled")) -> ()  [unwired: 1 in, 2 out]
                              }
                              frame True {
                                n288 = control-ref of="Det 2"() -> (w485:refnum<vi>)
                                n289 = property on="Property Node" class="Digital (strict)"(reference=w485, "DisabledEnum"=T4."Enabled" ("Disabled")) -> ()  [unwired: 1 in, 2 out]
                              }
                            }
                            n290 = case shown="True" w349 {
                              frame False {
                                n291 = control-ref of="Det 3"() -> (w479:refnum<vi>)
                                n292 = property on="Property Node" class="Digital (strict)"(reference=w479, "DisabledEnum"=T4."Disabled and Grayed Out" ("Disabled")) -> ()  [unwired: 1 in, 2 out]
                              }
                              frame True {
                                n293 = control-ref of="Det 3"() -> (w481:refnum<vi>)
                                n294 = property on="Property Node" class="Digital (strict)"(reference=w481, "DisabledEnum"=T4."Enabled" ("Disabled")) -> ()  [unwired: 1 in, 2 out]
                              }
                            }
                            n295 = case shown="True" w350 {
                              frame False {
                                n296 = control-ref of="Det 4"() -> (w475:refnum<vi>)
                                n297 = property on="Property Node" class="Digital (strict)"(reference=w475, "DisabledEnum"=T4."Disabled and Grayed Out" ("Disabled")) -> ()  [unwired: 1 in, 2 out]
                              }
                              frame True {
                                n298 = control-ref of="Det 4"() -> (w477:refnum<vi>)
                                n299 = property on="Property Node" class="Digital (strict)"(reference=w477, "DisabledEnum"=T4."Enabled" ("Disabled")) -> ()  [unwired: 1 in, 2 out]
                              }
                            }
                            n300 = case shown="True" w351 {
                              frame False {
                                n301 = control-ref of="Det 5"() -> (w471:refnum<vi>)
                                n302 = property on="Property Node" class="Digital (strict)"(reference=w471, "DisabledEnum"=T4."Disabled and Grayed Out" ("Disabled")) -> ()  [unwired: 1 in, 2 out]
                              }
                              frame True {
                                n303 = control-ref of="Det 5"() -> (w473:refnum<vi>)
                                n304 = property on="Property Node" class="Digital (strict)"(reference=w473, "DisabledEnum"=T4."Enabled" ("Disabled")) -> ()  [unwired: 1 in, 2 out]
                              }
                            }
                            n305 = case shown="False" w352 {
                              frame False {
                                n306 = control-ref of="Det 6"() -> (w467:refnum<vi>)
                                n307 = property on="Property Node" class="Digital (strict)"(reference=w467, "DisabledEnum"=T4."Disabled and Grayed Out" ("Disabled")) -> ()  [unwired: 1 in, 2 out]
                              }
                              frame True {
                                n308 = control-ref of="Det 6"() -> (w469:refnum<vi>)
                                n309 = property on="Property Node" class="Digital (strict)"(reference=w469, "DisabledEnum"=T4."Enabled" ("Disabled")) -> ()  [unwired: 1 in, 2 out]
                              }
                            }
                            n310 = case shown="True" w353 {
                              frame False {
                                n311 = control-ref of="Det 7"() -> (w463:refnum<vi>)
                                n312 = property on="Property Node" class="Digital (strict)"(reference=w463, "DisabledEnum"=T4."Disabled and Grayed Out" ("Disabled")) -> ()  [unwired: 1 in, 2 out]
                              }
                              frame True {
                                n313 = control-ref of="Det 7"() -> (w465:refnum<vi>)
                                n314 = property on="Property Node" class="Digital (strict)"(reference=w465, "DisabledEnum"=T4."Enabled" ("Disabled")) -> ()  [unwired: 1 in, 2 out]
                              }
                            }
                            n315 = case shown="True" w354 {
                              frame False {
                                n316 = control-ref of="Det 8"() -> (w459:refnum<vi>)
                                n317 = property on="Property Node" class="Digital (strict)"(reference=w459, "DisabledEnum"=T4."Disabled and Grayed Out" ("Disabled")) -> ()  [unwired: 1 in, 2 out]
                              }
                              frame True {
                                n318 = control-ref of="Det 8"() -> (w461:refnum<vi>)
                                n319 = property on="Property Node" class="Digital (strict)"(reference=w461, "DisabledEnum"=T4."Enabled" ("Disabled")) -> ()  [unwired: 1 in, 2 out]
                              }
                            }
                            n320 = Or(x=w421, y=w454) -> (x .or. y?=w452:bool)
                            n321 = case shown="True" w452 {
                              tunnel: w423 -> [w578 _]
                              frame True {
                                n322 = case shown="\"8 Detectors\", Default" w578 {
                                frame "4 Detectors" {
                                n323 = dll-call lib="C:/Users/BUCKLEY-ADMIN/Desktop/DCScode_simulISS_MAP/flex05-4chPascal.dll" fn="USBStop" label="StopCH4"() -> ()  [unwired: 4 in, 2 out]
                                }
                                frame "8 Detectors", Default {
                                n324 = dll-call lib="C:/Users/BUCKLEY-ADMIN/Desktop/DCScode_simulISS_MAP/flex05oem8chauto100nsPASCAL_win7.dll" fn="USBStop" label="StopCH8"() -> ()  [unwired: 4 in, 2 out]
                                }
                                }
                              }
                              frame False {
                              }
                            }
                          }
                          n325 = Current VI's Menubar() -> (w259:refnum<k9>)
                          n326 = local read "Trial #"() -> (w252:u32)
                          n327 = property on="QUIT" class="Bool"("Disabled"=w266) -> ()  [unwired: 2 in, 2 out]
                          n328 = Set Menu Item Info(7:"File", 9:w257, 11:w259) -> (3:w258:refnum<k9>)  [unwired: 4 in, 1 out]
                          n329 = Increment(x=w252) -> (x+1=w251:u32)
                          n330 = property on="Sequence Scan" class="Bool"("Disabled"=w266) -> ()  [unwired: 2 in, 2 out]
                          n331 = property on="Update Time (ms)\nDO NOT CHANGE!" class="DigNum (strict)"("Disabled"=w266) -> ()  [unwired: 2 in, 2 out]
                          n332 = property on="Integration Time (ms)" class="DigNum (strict)"("Disabled"=w266) -> ()  [unwired: 2 in, 2 out]
                          n333 = property on="Detector Select" class="RadioBtnsControl (strict)"("Disabled"=w266) -> ()  [unwired: 2 in, 2 out]
                          n334 = property on="Initialize Correlator" class="Bool"("Disabled"=w266) -> ()  [unwired: 2 in, 2 out]
                          n335 = local write "Trial #"(w251) -> ()
                          n336 = Set Menu Item Info(7:"Options", 9:w257, 11:w258) -> ()  [unwired: 4 in, 2 out]
                          n337 = case shown="\"Det 2\"" "Detector Used" {
                            tunnel: [1 2 3 4 5 6 7 8] -> w254
                            frame "Det 1", Default {
                            }
                            frame "Det 2" {
                            }
                            frame "Det 3" {
                            }
                            frame "Det 4" {
                            }
                            frame "Det 5" {
                            }
                            frame "Det 6" {
                            }
                            frame "Det 7" {
                            }
                            frame "Det 8" {
                            }
                          }
                          n338 = for {
                            N: 1 -> [_]
                            tunnel: w262 -> [w308]
                            tunnel: [w311] -> w255
                            tunnel: w254 -> [w310]
                            tunnel: w247 -> [w301]
                            n339 = case shown="True" w301 {
                              tunnel: [u32 0 w317] -> w311
                              frame False {
                              }
                              frame True {
                                n340 = local write "Trial #"(u32 0) -> ()
                                n341 = local read "Mark #"() -> (w319:u32)
                                n342 = Increment(x=w319) -> (x+1=w317:u32)
                                n343 = local write "Mark #"(w317) -> ()
                              }
                            }
                            n344 = Index Array(array=w308, index=w310) -> (element=w309:sgl)
                            n345 = Boolean To (0,1)(Boolean="Baseline") -> (0, 1=w313:i16)
                            n346 = case shown="False" w301 {
                              tunnel: [0.0 w315] -> w305
                              tunnel: inf -> [_ w315]
                              frame False {
                              }
                              frame True {
                              }
                            }
                            n347 = feedback #1() -> (w306:sgl)  [unwired: 1 in]
                            n348 = formula code="if(Tau==0) Tau=Tau+0.001;\nif(T==1) baselineflow=Tau;\n\ntmp=baselineflow/Tau;"("Tau"=w309, "T"=w313, "baselineflow"=w306) -> ("tmp"=w303:dbl, "baselineflow"=w307:sgl)
                            n349 = feedback-in #1(w307) -> ()
                            n350 = Bundle("tmp"=w303, w305) -> (→"Tau":cluster{"tmp":dbl, dbl})  [unwired: 1 in]
                          }
                          n351 = property on="Frame #" class="DigNum (strict)"() -> ("Value"=w238:u32)  [unwired: 2 in, 2 out]
                          n352 = case shown="True" "Fixed Time" {
                            tunnel: w238 -> [w289 w292]
                            tunnel: [w289 w292] -> w237
                            frame False {
                            }
                            frame True {
                              n353 = Less Or Equal?(x="Fixed # of Frames", y=w292) -> (x <= y?=w290:bool)
                              n354 = local write "Stop"(w290) -> ()
                            }
                          }
                          n355 = case shown="\"8 Detectors\", Default" w245 {
                            tunnel: w255 -> [w586 w590]
                            tunnel: [w587 w589] -> w272
                            tunnel: [4 8] -> w244
                            frame "4 Detectors" {
                              n356 = Build Array(w586, w586, w586, w586, w586) -> (w587:u32[])
                            }
                            frame "8 Detectors", Default {
                              n357 = Build Array(w590, w590, w590, w590, w590, w590, w590, w590, w590) -> (w589:u32[])
                            }
                          }
                          n358 = case shown="\"8 Detectors\", Default" w245 {
                            tunnel: ["%Duration\tID1\t\tID2\t\tID3\t\tID4\n" "%Duration\tID1\t\tID2\t\tID3\t\tID4\t\tID5\t\tID6\t\tID7\t\tID8\n"] -> w269
                            tunnel: ["%Tau\t\tTau1\t\tTau2\t\tTau3\t\tTau4\n" "%Tau\t\tTau1\t\tTau2\t\tTau3\t\tTau4\t\tTau5\t\tTau6\t\tTau7\t\tTau8\n"] -> w268
                            tunnel: ["%Delaytime\tD1\t\tD2\t\tD3\t\tD4\n" "%Delaytime\tD1\t\tD2\t\tD3\t\tD4\t\tD5\t\tD6\t\tD7\t\tD8\n"] -> w267
                            frame "4 Detectors" {
                            }
                            frame "8 Detectors", Default {
                            }
                          }
                          n359 = Increment(x=w237) -> (x+1=w239:u32)
                          n360 = Number To Decimal String(number=w237) -> (decimal integer string=w273:string)  [unwired: 1 in]
                          n361 = local write "Frame #"(w239) -> ()
                          n362 = Get Date/Time In Seconds() -> (seconds since 1Jan1904=w282:timestamp)
                          n363 = Array To Spreadsheet String(array=w272, 3:"%d") -> (spreadsheet string=w270:string)  [unwired: 1 in]
                          n364 = Format Date/Time String(seconds (now)=w282) -> (date/time string=w279:string)  [unwired: 2 in]
                          "Computer Time" <- w279
                          n365 = Concatenate Strings("File\nName:", "_flow_", w273, ".dat") -> (w242:string)
                          n366 = local read "Test"() -> (w236:bool)
                          n367 = Concatenate Strings("%", w279, "\r\n", w269, w265, w268, "%\t\t", w264, w267, w263, w270) -> (w250:string)
                          n368 = Build Path(base path="Data Save Directory:", name or relative path=w242) -> (appended path=w249:path)
                          n369 = case shown="False" w236 {
                            tunnel: w250 -> [w286 _]
                            tunnel: w249 -> [w285 _]
                            tunnel: [w284 _] -> w248
                            tunnel: [w283 _] -> w246
                            frame False {
                              n370 = Write to Text File(file (use dialog)=w285, text=w286) -> (refnum out=w287:refnum<file>, error out=w288:errorcluster)  [unwired: 2 in, 1 out]
                              n371 = Close File(refnum=w287, error in=w288) -> (path=w284:path, error out=w283:errorcluster)
                            }
                            frame True {
                            }
                          }
                        }
                      }
                      n372 = Index Array(array="Visible Averages", index=3) -> (element=w185:bool)
                      n373 = Index Array(array="Visible Averages", index=1) -> (element=w186:bool)
                      n374 = Index Array(array="Visible Averages", index=0) -> (element=w179:bool)
                      n375 = Index Array(array="Visible Averages", index=2) -> (element=w180:bool)
                      n376 = property on="Tau 2" class="WFChart (strict)"("Active Plot"=u32 11) -> (error out=w183:errorcluster)  [unwired: 2 in, 1 out]
                      n377 = property on="Tau 2" class="WFChart (strict)"("Active Plot"=u32 9) -> (error out=w188:errorcluster)  [unwired: 2 in, 1 out]
                      n378 = property on="Tau 2" class="WFChart (strict)"("Active Plot"=u32 8) -> (error out=w177:errorcluster)  [unwired: 2 in, 1 out]
                      n379 = property on="Tau 2" class="WFChart (strict)"("Active Plot"=u32 10) -> (error out=w182:errorcluster)  [unwired: 2 in, 1 out]
                      n380 = property on="Tau 2" class="WFChart (strict)"(error in=w183, "Plot.Visible?"=w185) -> ()  [unwired: 1 in, 2 out]
                      n381 = property on="Tau 2" class="WFChart (strict)"(error in=w188, "Plot.Visible?"=w186) -> ()  [unwired: 1 in, 2 out]
                      n382 = property on="Tau 2" class="WFChart (strict)"(error in=w177, "Plot.Visible?"=w179) -> ()  [unwired: 1 in, 2 out]
                      n383 = property on="Tau 2" class="WFChart (strict)"(error in=w182, "Plot.Visible?"=w180) -> ()  [unwired: 1 in, 2 out]
                      n384 = local read "Test"() -> (w163:bool)
                      n385 = Not(x=w163) -> (.not. x?=w162:bool)
                      n386 = Unbundle By Name(w171) -> ("status"=w190:bool)
                      n387 = for {
                        N: 1 -> [_]
                        tunnel: w191 -> [_]
                        n388 = local write "Stop"(FALSE) -> ()
                        n389 = Wait (ms)(milliseconds to wait="Delay between frames(ms)") -> ()  [unwired: 1 out]
                      }
                      n390 = And(x="Real Time Fitting?", y=w162) -> (x .and. y?=w161:bool)
                      n391 = Not(x=w190) -> (.not. x?=w189:bool)
                      n392 = case shown="True" w161 {
                        tunnel: w189 -> [_ w200]
                        tunnel: w170 -> [_ w199]
                        tunnel: w169 -> [_ w198]
                        tunnel: w166 -> [w195 w197]
                        tunnel: [w195 w196] -> w165
                        frame False {
                        }
                        frame True {
                          n393 = case shown="True" w200 {
                            tunnel: w199 -> [_ w220]
                            tunnel: w198 -> [_ w216]
                            tunnel: w197 -> [w201 w212]
                            tunnel: [w201 w210] -> w196
                            frame False {
                            }
                            frame True {
                              # "Initialize Array of NaNs with size of \"fixed number of frames, \nand run this array into the case structure by putting it \nthrough a shift register with each loop it will replace one of \nthe NaNs by the flow data of the detector used. Then this data\nis averaged and COV is calculated."
                              n394 = property on="Data Save Directory:" class="Path"() -> ("Value"=w222:path)  [unwired: 2 in, 2 out]
                              n395 = property on="File\nName:" class="Str"() -> ("Value"=w223:string)  [unwired: 2 in, 2 out]
                              n396 = call "GetFilePath.vi"("path"=w222, "file name"=w223, "frame number"=w220) -> ("final path C"=w215:string)  [unwired: 10 in, 2 out]
                              n397 = property on="Avg" class="Arr (strict)"() -> ("Value"=w221:bool[][])  [unwired: 2 in, 2 out]
                              n398 = call "DCSAnalysis.vi"("# Detectors"=w216, "File path"=w215, "Frame #"=w220, "rho"="rho", "other settings"="Other Settings", "avgBool"=w221, "var values"="Initial Guess") -> ("Flow in each detector"=w213:dbl[], "Tau"=→"Tau 2":T3)  [unwired: 18 in, 1 out]
                              "Flow in each detector" <- w213
                              n399 = local read "Detector Used"() -> (w202:T2)
                              n400 = local read "Trial #"() -> (w208:u32)
                              n401 = Decrement(x=w208) -> (x-1=w209:u32)
                              n402 = Index Array(array=w213, index=w202) -> (element=w211:dbl)
                              n403 = Replace Array Subset(array=w212, new element=w211, index=w209) -> (w210:dbl[])
                              n404 = call <vilib>:"Std Deviation and Variance.vi"("X"=w210) -> ("mean"=w206:dbl, "standard deviation"=w207:dbl)  [unwired: 1 in, 1 out]
                              "mean" <- w206
                              n405 = Divide(x=w207, y=w206) -> (x/y=w204:dbl)
                              n406 = Multiply(x=w204, y=100.0) -> (x*y=→"COV":dbl)
                            }
                          }
                        }
                      }
                    }
                    n407 = call "iBs.vi"("Laser On/Off"=TRUE, "VISA resource name"="Laser Input Name") -> ()
                  }
                  frame True {
                    n408 = invoke on="Sequence Scan" class="Bool" method="Reinit To Default"() -> ()  [unwired: 3 in, 3 out]
                    n409 = call "Display Message to User5"() -> ()  [unwired: 10 in, 2 out]
                  }
                }
              }
            }
            "Frame #" <- u32 0
            "Mark #" <- u32 0
            "Trial #" <- u32 0
          }
          event "QUIT": Value Change {
            # "Reset correlator before quitting"
            n410 = event-data() -> ()  [unwired: 1 in, 6 out]
            n411 = case shown="\"8 Detectors\", Default" w598 {
              frame "4 Detectors" {
                n412 = dll-call lib="C:/Users/BUCKLEY-ADMIN/Desktop/DCScode_simulISS_MAP/flex05-4chPascal.dll" fn="USBInitialize" label="InitCH4"() -> (error out=w600:errorcluster)  [unwired: 4 in, 1 out]
                n413 = dll-call lib="C:/Users/BUCKLEY-ADMIN/Desktop/DCScode_simulISS_MAP/flex05-4chPascal.dll" fn="USBFree" label="FreeCH4"(error in=w600) -> ()  [unwired: 3 in, 2 out]
              }
              frame "8 Detectors", Default {
                n414 = dll-call lib="C:/Users/BUCKLEY-ADMIN/Desktop/DCScode_simulISS_MAP/flex05oem8chauto100nsPASCAL_win7.dll" fn="USBInitialize" label="InitCH8"() -> (error out=w601:errorcluster)  [unwired: 4 in, 1 out]
                n415 = dll-call lib="C:/Users/BUCKLEY-ADMIN/Desktop/DCScode_simulISS_MAP/flex05oem8chauto100nsPASCAL_win7.dll" fn="USBFree" label="FreeCH8"(error in=w601) -> ()  [unwired: 3 in, 2 out]
              }
            }
            n416 = local write "Status"("Quit") -> ()
            n417 = local write "Status"("Quit") -> ()
          }
          event Timeout {
            w606 = TRUE
            w605 = u8 0
            # "This case structure turns on\n      and off the ISS Lasers"
            # "This case structure ensures that when the\noptical switch is turned on, the relay tells \nthe laser to power on."
            # "The system sits here and wait for some buttons to be pressed. And the status is always \"waiting\". Once some button is pressed, this value driven event\nstructure goes to the appropriate frame."
            n418 = event-data() -> ()  [unwired: 1 in, 3 out]
            n419 = local write "Status"("Waiting") -> ()
            n420 = property on="MARK\nMark" class="Bool"("DisabledEnum"=w605) -> ()  [unwired: 2 in, 2 out]
            n421 = property on="QUIT" class="Bool"("Disabled"=w605) -> ()  [unwired: 2 in, 2 out]
            n422 = property on="Sequence Scan" class="Bool"("Disabled"=w605) -> ()  [unwired: 2 in, 2 out]
            n423 = property on="Initialize Correlator" class="Bool"("Disabled"=w605) -> ()  [unwired: 2 in, 2 out]
            n424 = property on="Update Time (ms)\nDO NOT CHANGE!" class="DigNum (strict)"("Disabled"=w605) -> ()  [unwired: 2 in, 2 out]
            n425 = property on="Integration Time (ms)" class="DigNum (strict)"("Disabled"=w605) -> ()  [unwired: 2 in, 2 out]
            n426 = property on="Detector Select" class="RadioBtnsControl (strict)"("Disabled"=w605) -> ()  [unwired: 2 in, 2 out]
            n427 = case shown="True" "ISS Lasers ON" {
              frame False {
                n428 = Build Array(FALSE) -> (w613:bool[])
                n429 = call "DAQ Assistant5"("data"=w613) -> ()  [unwired: 17 in, 2 out]
              }
              frame True {
                # "For Toptica laser control"
                n430 = local read "Laser Input Name"() -> (w615:refnum<visa-resource-name>)
                n431 = call "iBs.vi"("Laser On/Off"=TRUE, "VISA resource name"=w615) -> ()
                n432 = Build Array(TRUE) -> (w617:bool[])
                n433 = call "DAQ Assistant6"("data"=w617) -> ()  [unwired: 17 in, 2 out]
              }
            }
            n434 = case shown="True" "Optical Switch OPEN" {
              frame False {
                # "Send 2 signals, one for LED indicator, one for switch"
                n435 = Build Array(FALSE, FALSE) -> (w619:bool[])
                n436 = call "DAQ Assistant3"("data"=w619) -> ()  [unwired: 17 in, 2 out]
              }
              frame True {
                n437 = Build Array(TRUE, TRUE) -> (w622:bool[])
                n438 = call "DAQ Assistant4"("data"=w622) -> ()  [unwired: 17 in, 2 out]
              }
            }
            n439 = Current VI's Menubar() -> (w608:refnum<k9>)
            n440 = Set Menu Item Info(7:"File", 9:w606, 11:w608) -> (3:w607:refnum<k9>)  [unwired: 4 in, 1 out]
            n441 = Get Date/Time In Seconds() -> (seconds since 1Jan1904=w611:timestamp)
            n442 = Set Menu Item Info(7:"Options", 9:w606, 11:w607) -> ()  [unwired: 4 in, 2 out]
            n443 = Format Date/Time String(seconds (now)=w611) -> (date/time string=w612:string)  [unwired: 2 in]
            n444 = local write "Computer Time"(w612) -> ()
          }
        }
      }
    }
  }
